vi "obtain_latest_instance.vi"(7 "quick, but maybe outdated?":bool=TRUE, 8 "error in (no error)":errorcluster) -> (0 "error out":errorcluster, 3 "GeneralAnalyser out":refnum<class "GenericAnalyser.lvclass">)   [LabVIEW 2010, in "GenericAnalyser.lvclass"]
uses:
  GenericAnalyser.lvclass
  common/classes/ErrorController/ErrorController/class_data.vi
  class_data.vi
  common/classes/ErrorController/ErrorController/ErrorController.lvclass
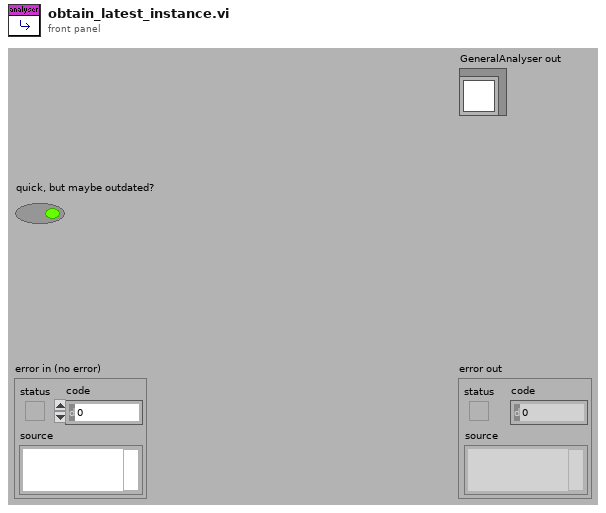
[diagram p1: front panel]
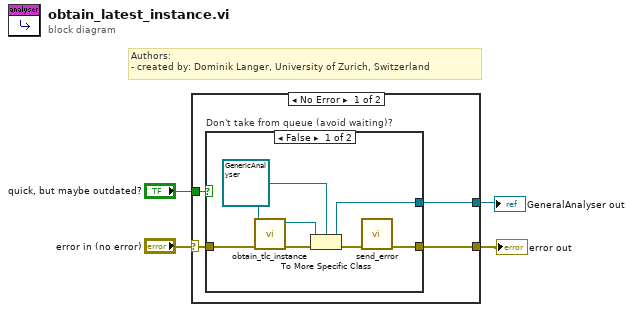
[diagram p0: block diagram]
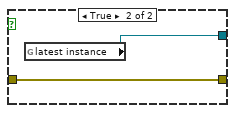
[diagram p2: hidden frame]
diagram:
  # "Authors: \n- created by: Dominik Langer, University of Zurich, Switzerland"
  n1 = case shown="No Error" "error in (no error)" {
    selector: "error in (no error)" -> [w8 w18]
    tunnel: [w7 w18] -> w3
    tunnel: "quick, but maybe outdated?" -> [w6 _]
    tunnel: [w5 _] -> w1
    frame No Error {
      n2 = case "Don't take from queue (avoid waiting)?" shown="False" w6 {
        tunnel: w8 -> [w12 w17]
        tunnel: [w10 w17] -> w7
        tunnel: [w13 w16] -> w5
        frame False {
          w9 = refnum<class "GenericAnalyser.lvclass"> refnum ("GeneralAnalyser.lvclass")
          n3 = call-dynamic "obtain_tlc_instance.vi"("error in (no error)"=w12, "GenericToplevelComponent in"=w9) -> ("error out"=w15:errorcluster, "GenericToplevelComponent out"=w14:refnum<class "GenericToplevelComponent.lvclass">)  [unwired: 8 in]
          n4 = To More Specific Class(target class=w9, reference=w14, error in=w15) -> (specific class reference=w13:refnum<class "GenericAnalyser.lvclass">, error out=w11:errorcluster)
          n5 = call "send_error.vi"("error in (no error)"=w11) -> ("error out"=w10:errorcluster)  [unwired: 10 in]
        }
        frame True {
          n6 = global read "class_data.vi" "latest instance"() -> (w16:refnum<class "GenericAnalyser.lvclass">)
        }
      }
    }
    frame Error {
    }
  }
  "error out" <- w3
  "GeneralAnalyser out" <- w1
